vi "MotorOnOff.vi"(7 "#Axis":i32, 8 "error in":errorcluster, 10 "Enabled":bool, 11 "VISA resource":refnum<visa-resource-name>) -> (0 "error out":errorcluster)   [LabVIEW 2014, in "GRBLMotionCore.lvlib"]
uses:
  <instrlib>/GRBL/GRBLMotionCore.lvlib
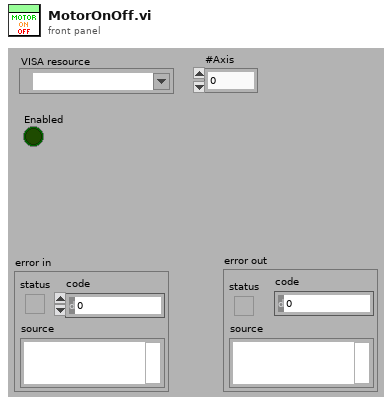
[diagram p1: front panel]
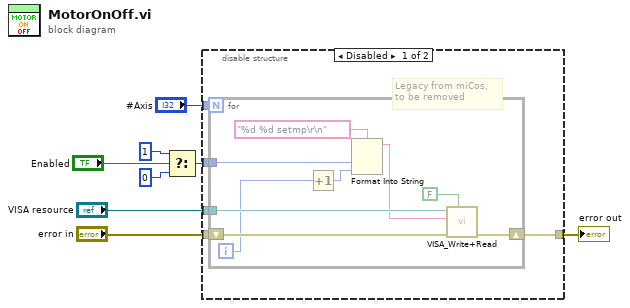
[diagram p0: block diagram]
diagram:
  n1 = Select(t=i8 1, s="Enabled", f=i8 0) -> (s? t:f=w4:i8)
  n2 = disable-structure shown="Disabled" {
    disable-tunnel: "VISA resource" -> [w13 _]
    disable-tunnel: "error in" -> [w12 w23]
    disable-tunnel: [w11 w23] -> w6
    disable-tunnel: w4 -> [w10 _]
    disable-tunnel: "#Axis" -> [w9 _]
    frame Disabled {
      # "Legacy from miCos,\nto be removed"
      n3 = for {
        N: w9 -> [_]
        tunnel: w13 -> [w22]
        tunnel: w10 -> [w19]
        shift-right: [w20] -> w11
        shift-left: w12 -> [w21]
        i -> [w15]
        n4 = Increment(x=w15) -> (x+1=w16:i32)
        n5 = Format Into String(format string="%d %d setmp\r\n", w19, w16) -> (resulting string=w14:string)  [unwired: 2 in, 1 out]
        n6 = call <instrlib>:"VISA_Write+Read.vi"("Read? (T)"=FALSE ("Read?"), "error in (no error)"=w21, "Write Buffer"=w14, "VISA resource name"=w22) -> ("error out"=w20:errorcluster)  [unwired: 5 in, 2 out]
      }
    }
    frame Enabled {
    }
  }
  "error out" <- w6
